vi "String Empty.vi"(1 "String":string) -> (0 "Empty?":bool)   [LabVIEW 2011]
doc: "Returns T if string is empty/null.\n\n\nVersion 1.0 - 2/20/2012\n\nPhaeron, Inc.\nwww.phaeron.com\ninfo@phaeron.com"
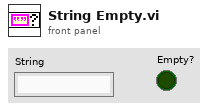
[diagram p1: front panel]
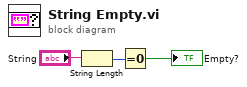
[diagram p0: block diagram]
diagram:
  n1 = String Length(string="String") -> (length=w2:i32)
  n2 = Equal To 0?(x=w2) -> (x = 0?=→"Empty?":bool)
